vi "create.vi"(8 "error in (no error)":errorcluster, 11 "GenericStringGenerator in":refnum<class "GenericStringGenerator.lvclass">) -> (0 "error out":errorcluster, 2 "String":string, 3 "GenericStringGenerator out":refnum<class "GenericStringGenerator.lvclass">)   [LabVIEW 2010, in "GenericStringGenerator.lvclass"]
uses:
  GenericStringGenerator.lvclass
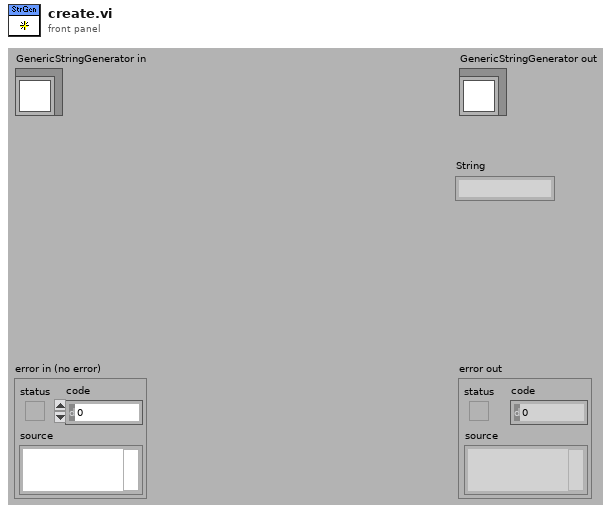
[diagram p1: front panel]
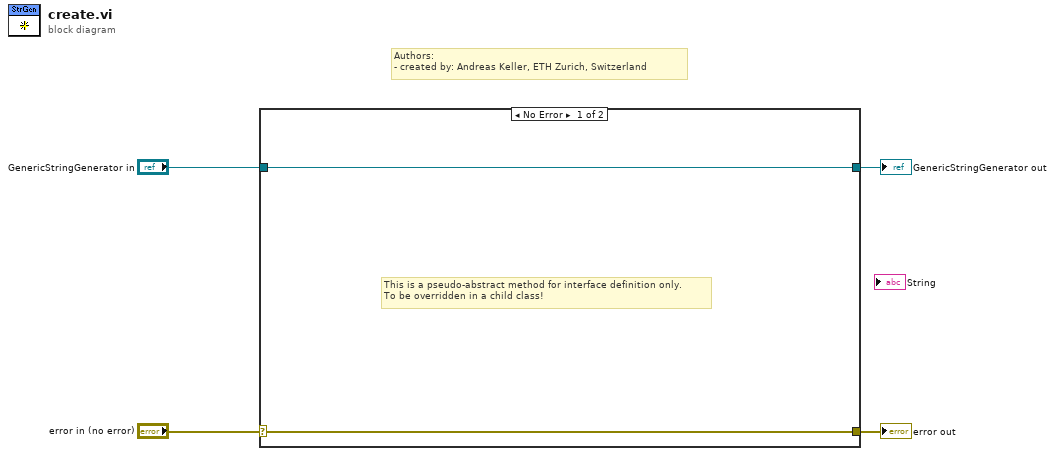
[diagram p0: block diagram]
diagram:
  # "Authors: \n- created by: Andreas Keller, ETH Zurich, Switzerland"
  n1 = case shown="No Error" "error in (no error)" {
    selector: "error in (no error)" -> [w6 w8]
    tunnel: [w6 w8] -> w3
    tunnel: [w5 w7] -> w1
    tunnel: "GenericStringGenerator in" -> [w5 w7]
    frame No Error {
      # "This is a pseudo-abstract method for interface definition only.\nTo be overridden in a child class!"
    }
    frame Error {
    }
  }
  "error out" <- w3
  "GenericStringGenerator out" <- w1
